vi "SMU.Keithley2600.ReftoDVR.vi"(10 "Ref":u32 format="%08x") -> (2 "Ref":T1)   [LabVIEW 2017, in "SMU.Keithley2600.lvclass"]
doc: "JKI State Machine Objects (SMO) 1.0.0.5\nJKI - JKI\nCopyright (c) 2016, JKI"
uses:
  SMU.Keithley2600.lvclass
  Typedefs/PrivateData--Ref.ctl
  Typedefs/PrivateData--Cluster.ctl
  Typedefs/Resource--Cluster.ctl
  <instrlib>/Keithley 2600 Series/Public/Channel.ctl
  <instrlib>/Keithley 2600 Series/Keithley 2600 Series.lvlib
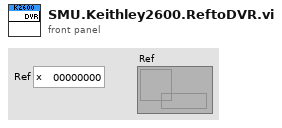
[diagram p1: front panel]
types:
  T1 = typedef "SMU.Keithley2600.lvclass/PrivateData--Ref.ctl" = refnum<data-value>
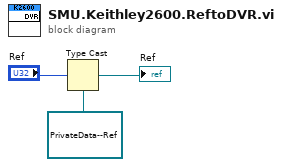
[diagram p0: block diagram]
diagram:
  n1 = Type Cast(type=T1 refnum ("Ref"), x="Ref") -> (*(type *) &x=→"Ref":T1)
